vi "test_LoadFrameEditorFile.vi"(11 "file path (use dialog)":path) -> (0 "error out":errorcluster, 3 "data":T4[](array[typedef]) {"value"."Data" format="%.0x"; "value"."HeaderInfo"."NetSelect" items=["FDX_TX_FRAME_DLY_A"=0, "FDX_TX_FRAME_DLY_B"=1, "FDX_TX_FRAME_BOTH "=3, "FDX_TX_FRAME_ONLY_A"=4, "FDX_TX_FRAME_ONLY_B "=5]; "value"."HeaderInfo"."FrameStartMode" items=["FDX_TX_FRAME_START_IFG", "FDX_TX_FRAME_START_PGWT", "FDX_TX_FRAME_START_TRG"]; "value"."HeaderInfo"."PhysErrorInjection" items=["FDX_TX_FRAME_ERR_OFF"=0, "FDX_TX_FRAME_ERR_CRC"=1, "FDX_TX_FRAME_ERR_ALI"=2, "FDX_TX_FRAME_ERR_PRE"=4, "FDX_TX_FRAME_ERR_PHY"=8]; "value"."HeaderInfo"."SequenceNumberInit" items=["FDX_TX_FRAME_SEQ_INIT_AUTO"=65535]; "value"."HeaderInfo"."SequenceNumberOffset" items=["FDX_TX_FRAME_SEQ_OFFS_AUTO "=65535]; "value"."HeaderInfo"."PayloadGenerationMode" items=["FDX_TX_FRAME_PGM_USER"=0, "FDX_TX_FRAME_PGM_IP_PART"=1, "FDX_TX_FRAME_PGM_IP_FULL"=2, "FDX_TX_FRAME_PGM_IP_PART_TT"=10, "FDX_TX_FRAME_PGM_IP_FULL_TT"=20]; "value"."HeaderInfo"."PayloadBufferMode" items=["FDX_TX_FRAME_PBM_STD", "FDX_TX_FRAME_PBM_MAC", "FDX_TX_FRAME_PBM_UDP"]})   [LabVIEW 2020]
uses:
  Frame Configuration/controls/frame_file_entry.ctl
  Frame Configuration/controls/frame_record_type.ctl
  <instrlib>/AIM GmbH/_AIM 664/_controls/queue_header_generic.ctl
  <instrlib>/AIM GmbH/_AIM 664/helpers/EthFrameManagement/controls/ehternetFrame_type.ctl
  <instrlib>/AIM GmbH/_AIM 664/helpers/EthFrameManagement/controls/IPFrame_type.ctl
  <instrlib>/AIM GmbH/_AIM 664/helpers/EthFrameManagement/controls/UDPFrame_type.ctl
  <instrlib>/AIM GmbH/_AIM 664/AIM664LV.lvlib
  <instrlib>/AIM GmbH/_AIM 664/helpers/EthFrameManagement/EthFrameManagement.lvlib
panel:
  out "dst ip":string
  out "src ip":string
  out "size(s)":i32
  out "UDP header":T1
  out "IP header":T2 {"CtlFlags" format="%.0b"; "Dest IP" format="%.0x"; "Source IP" format="%.0x"; "Checksum" format="%.0x"; "TTL" format="%.0x"; "FragOffset" format="%.0x"; "ID" format="%.0x"; "Length" format="%.0x"; "ToS" format="%.0x"; "IHL" format="%.0x"; "Version" format="%.0x"}
  out "UDP Header Only":u8[](array[numeric])
  out "IP Header Only":u8[](array[numeric]) format="%.0x"
  out "Ethernet header":T3 {"EtherType" format="%04x"; "Src MAC" format="%02x"; "Dest MAC" format="%.0b"}
  out "MAC Header Only":u8[](array[numeric]) format="%.0x"
  out "payload":u8[](array[numeric]) format="%.0x"
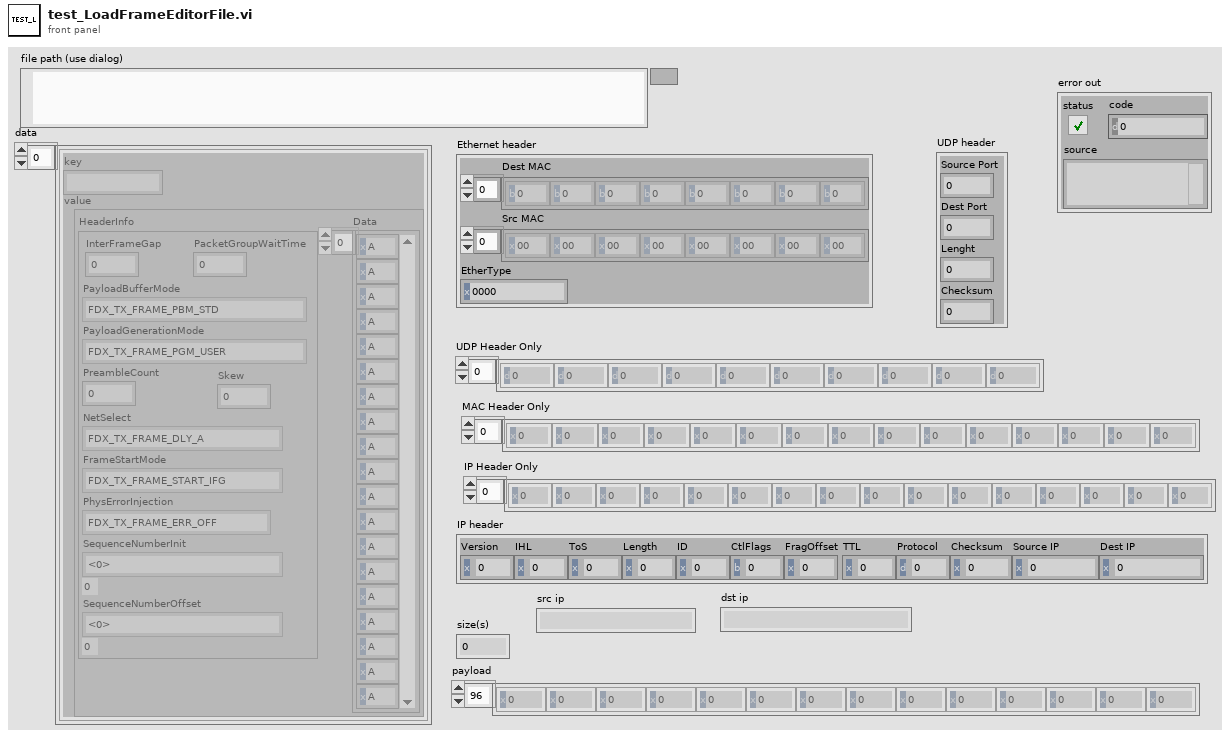
[diagram p1: front panel]
types:
  T1 = typedef "EthFrameManagement.lvlib/UDPFrame_type.ctl" = cluster{"Source Port":u16, "Dest Port":u16, "Lenght":u16, "Checksum":u16}
  T2 = typedef "EthFrameManagement.lvlib/IPFrame_type.ctl" = cluster{"Version":u8, "IHL":u8, "ToS":u8, "Length":u16, "ID":u16, "CtlFlags":u8, "FragOffset":u16, "TTL":u8, "Protocol":u8, "Checksum":u16, "Source IP":u32, "Dest IP":u32}
  T3 = typedef "EthFrameManagement.lvlib/ehternetFrame_type.ctl" = cluster{"Dest MAC":u8[], "Src MAC":u8[], "EtherType":u16}
  T4 = typedef "frame_file_entry.ctl" = cluster{"key":string, "value":T5}
  T5 = typedef "frame_record_type.ctl" = cluster{"HeaderInfo":T6, "Data":u8[]}
  T6 = typedef "AIM664LV.lvlib/queue_header_generic.ctl" = cluster{"InterFrameGap":u32, "PacketGroupWaitTime":u32, "PayloadBufferMode":u8, "PayloadGenerationMode":u8, "PreambleCount":u8, "Skew":u32, "NetSelect":u8, "FrameStartMode":u8, "PhysErrorInjection":u32, "SequenceNumberInit":u16, "SequenceNumberOffset":u16}
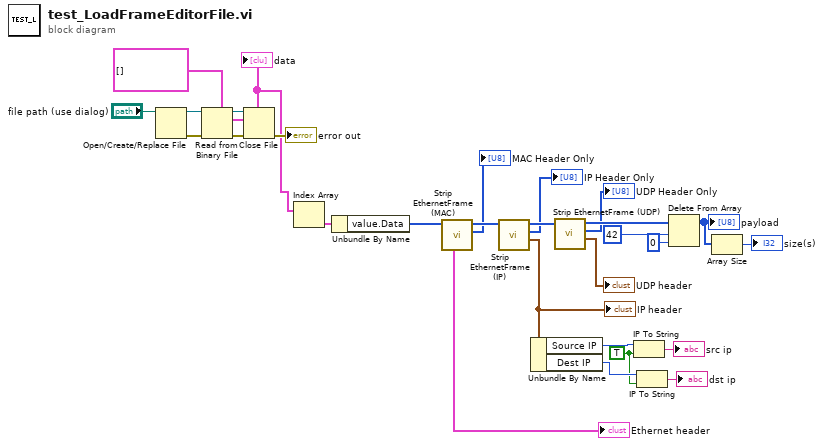
[diagram p0: block diagram]
diagram:
  w3 = TRUE ("dot notation? (F)")
  n1 = Open/Create/Replace File(file path (use dialog)="file path (use dialog)") -> (refnum out=w25:refnum<file>, error out=w24:errorcluster)  [unwired: 5 in, 1 out]
  n2 = Read from Binary File(5:T4[] [] ("cluster"), 8:w24, 11:w25) -> (0:w26:errorcluster, 2:w21:T4[], 3:w27:refnum<file>)  [unwired: 3 in, 1 out]
  "data" <- w21
  n3 = Close File(refnum=w27, error in=w26) -> (error out=→"error out":errorcluster)  [unwired: 1 out]
  n4 = Index Array(array=w21) -> (element=w20:T4)  [unwired: 1 in]
  n5 = Unbundle By Name(w20) -> ("value.Data"=w19:u8[])
  n6 = call <instrlib>:"Strip EthernetFrame (MAC).vi"("Ethernet Frame In"=w19) -> ("Ethernet header"=→"Ethernet header":T3, "MAC Header Only"=→"MAC Header Only":u8[], "Ethernet Frame Out"=w18:u8[])  [unwired: 7 in, 1 out]
  n7 = call <instrlib>:"Strip EthernetFrame (IP).vi"("Frame In"=w18) -> ("IP header"=w6:T2, "IP Header Only"=→"IP Header Only":u8[], "Frame Out"=w17:u8[])  [unwired: 7 in, 1 out]
  "IP header" <- w6
  n8 = Unbundle By Name(w6) -> ("Source IP"=w5:u32, "Dest IP"=w4:u32)
  n9 = call <instrlib>:"Strip EthernetFrame (UDP).vi"("Ethernet Frame In"=w17) -> ("UDP header"=→"UDP header":T1, "UDP Header Only"=→"UDP Header Only":u8[], "Ethernet Frame Out"=w16:u8[])  [unwired: 7 in, 1 out]
  n10 = IP To String(1:w3, 2:w5) -> (0:→"src ip":string)
  n11 = IP To String(1:w3, 2:w4) -> (0:→"dst ip":string)
  n12 = Delete From Array(array=w16, length=42 ("index"), index=0) -> (array with subset deleted=w8:u8[])  [unwired: 1 out]
  "payload" <- w8
  n13 = Array Size(array=w8) -> (size(s)=→"size(s)":i32)
